vi "API String - Set Float Precision.vi"(8 "Error in":errorcluster caption="Error in (no error)", 11 "Precision":u8=6) -> (0 "Error out":errorcluster, 3 "Float Format String":string)   [LabVIEW 2017, in "API String Arguments Support.lvlib"]
doc: "Sets the precision for floating-point numbers.\n\n> [!NOTE]\n> - The default precision is 6 significant digits, with the format `%.6p`.\n> - This VI is a simplified version of the API String - Set Float Format String VI, used only for setting the number of significant digits.\n\n\n> [!NOTE] <b>Default Floating-point Format</b>\n>\n> The default floating-point format is `%.6p`.\n\n\n-- <b>Controls</b> --\n- <b>Precision</b>: Floating-point precision setting.\n\n-- <b>Indicators</b> --\n- <b>Float Format String</b>: Updated floating-point format string."
uses:
  API String Arguments Support.lvlib
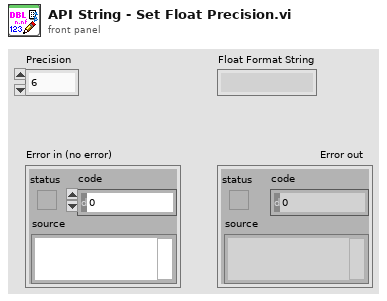
[diagram p1: front panel]
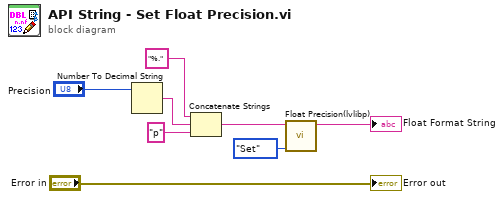
[diagram p0: block diagram]
diagram:
  n1 = Number To Decimal String(number="Precision") -> (decimal integer string=w6:string)  [unwired: 1 in]
  n2 = Concatenate Strings("%." ("format string"), w6, "p" ("format string")) -> (w2:string)
  n3 = call "Float Precision(lvlibp).vi"("Enum"=enum16{"Set", "Get"}."Set", "Precision"=w2) -> ("Format String"=→"Float Format String":string)  [unwired: 9 in]
  "Error out" <- "Error in"
